vi "Handle Error.vi"(7 "Stop on Unhandled Error (T)":bool=TRUE, 8 "error in":errorcluster, 11 "SMO":refnum<class "SMO.lvclass">) -> (0 "handling error":errorcluster, 2 "Unhandled error":errorcluster, 3 "SMO out":refnum<class "SMO.lvclass">)   [LabVIEW 2021, in "smo.lvlib" / "SMO.lvclass"]
doc: "JKI State Machine Objects (SMO) 1.0.0.11\nJKI - JKI\nCopyright (c) 2016, JKI"
uses:
  SMO.lvclass
  SMO.lvclass/SMO.ctl
  Private/ReftoDVR--SMO.vi
panel:
  # "For instructions on how to use the JKI State Machine Objects, examples and video tutorials, visit:\nhttp://jki.net/state-machine-objects/\n\nJKI State Machine Objects™\nhttp://jki.net/state-machine-objects/\nCopyright (C) 2005-2015, JKI <info@jki.net>\nALL RIGHTS RESERVED"
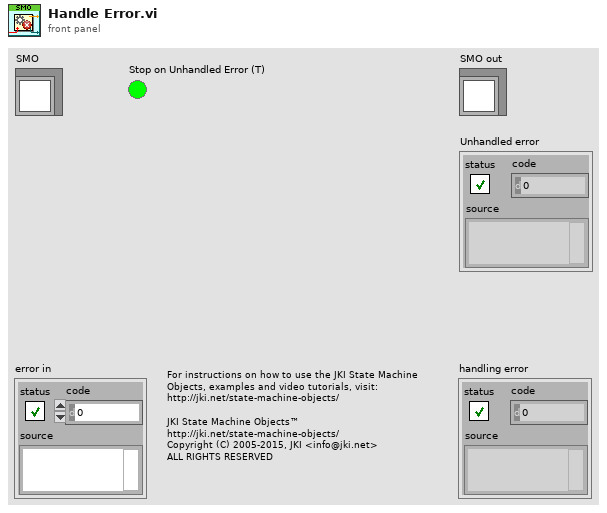
[diagram p1: front panel]
types:
  T1 = typedef "smo.lvlib/SMO.lvclass/Public Events.ctl" = cluster{"Error":refnum<user-event>, "State":refnum<user-event>, "Reserve State":refnum<user-event>}
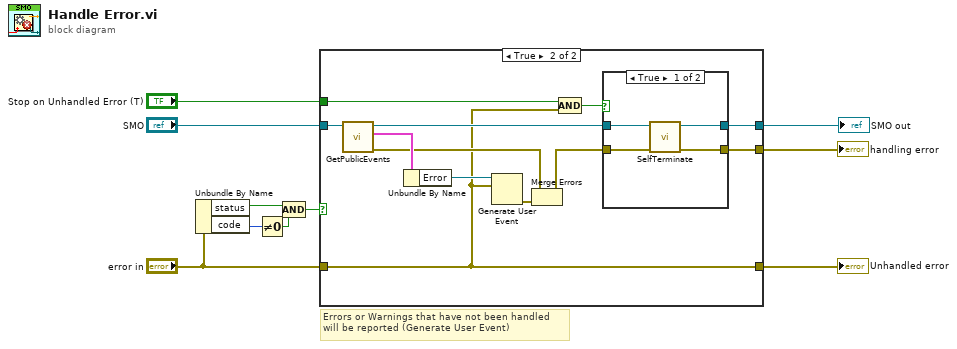
[diagram p0: block diagram]
diagram:
  # "Errors or Warnings that have not been handled\nwill be reported (Generate User Event)"
  n1 = Unbundle By Name("error in") -> ("status"=w8:bool, "code"=w7:i32)
  n2 = Not Equal To 0?(x=w7) -> (x != 0?=w5:bool)
  n3 = Compound Arithmetic op=AND(w8, w5) -> (w6:bool)
  n4 = case shown="True" w6 {
    tunnel: "SMO" -> [w12 w24]
    tunnel: [w12 w19] -> w10
    tunnel: [_ w16] -> w9
    tunnel: "error in" -> [w11 w15]
    tunnel: [w11 w15] -> w2
    tunnel: "Stop on Unhandled Error (T)" -> [_ w14]
    frame False {
    }
    frame True {
      n5 = call "GetPublicEvents.vi"("SMO"=w24) -> ("error out"=w21:errorcluster, "Public Events"=w23:T1, "SMO out"=w18:refnum<class "SMO.lvclass">)  [unwired: 8 in]
      n6 = Unbundle By Name(w23) -> ("Error"=w22:refnum<user-event>)
      n7 = Generate User Event(user event=w22, event data cluster=w15) -> (error out=w20:errorcluster)  [unwired: 2 in, 1 out]
      n8 = Merge Errors(w21, w20) -> (w17:errorcluster)
      n9 = Compound Arithmetic op=AND(w14, w15) -> (w13:bool)
      n10 = case shown="True" w13 {
        tunnel: [w27 w30] -> w19
        tunnel: w18 -> [w28 w30]
        tunnel: w17 -> [w26 w29]
        tunnel: [w25 w29] -> w16
        frame True {
          n11 = call "SelfTerminate.vi"("error in (no error)"=w26, "SMO in"=w28) -> ("error out"=w25:errorcluster, "SMO out"=w27:refnum<class "SMO.lvclass">)  [unwired: 8 in]
        }
        frame False {
        }
      }
    }
  }
  "handling error" <- w9
  "SMO out" <- w10
  "Unhandled error" <- w2
